vi "PI_GCS3_Configuration_Setup_Limits.vi"(0 "System no.":i32=1 min=1 step=1, 1 "Conn. Axes":string[](array[string]), 5 "error in":errorcluster) -> (14 "Positive Limit":dbl[](array[numeric]) format="%.6f", 16 "Negative Limit":dbl[](array[numeric]) format="%.6f", 19 "error out":errorcluster)   [LabVIEW 2026]
doc: "Gather positive and negative axes limits."
uses:
  SpecialCommand/ConfigurationMemoryType.ctl
panel:
  # "Gather positive and negative axes limits."
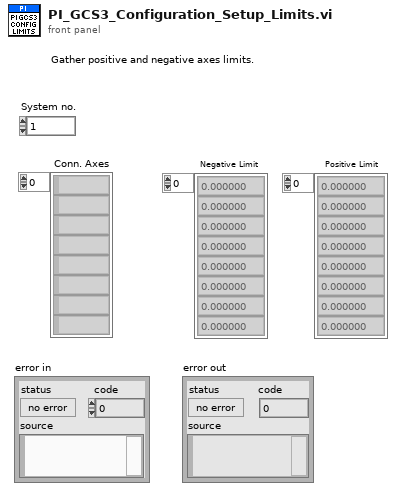
[diagram p1: front panel]
types:
  T1 = typedef "ConfigurationMemoryType.ctl" = enum16{"RAM", "TMP", "FLASH"}
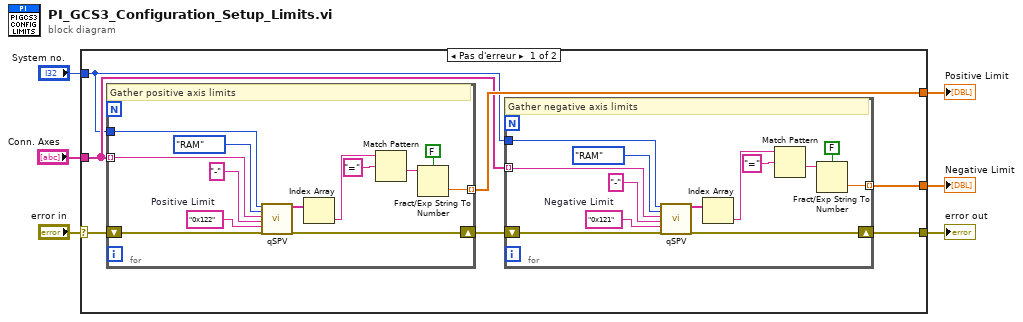
[diagram p0: block diagram]
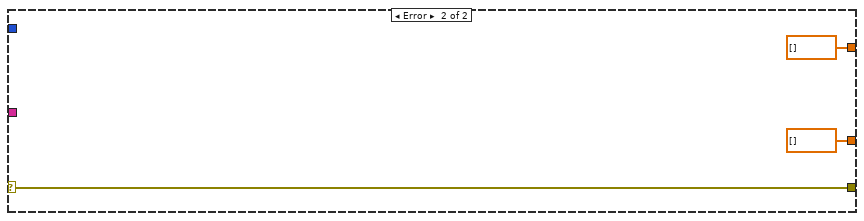
[diagram p2: hidden frame]
diagram:
  n1 = case shown="Pas d'erreur" "error in" {
    selector: "error in" -> [w13 w42]
    tunnel: [w8 w42] -> w5
    tunnel: "Conn. Axes" -> [w10 _]
    tunnel: "System no." -> [w9 _]
    tunnel: [w7 dbl[] [] ("Negative Limit")] -> w2
    tunnel: [w12 dbl[] [] ("Negative Limit")] -> w1
    frame No Error {
      n2 = for {
        shift-right: [w39] -> w11
        shift-left: w13 -> [w33]
        tunnel: w9 -> [w35]
        tunnel: w10 -> [w37] mode=indexing
        tunnel: [w32] -> w12 mode=indexing
        w38 = "0x122"  # Positive Limit
        # "Gather positive axis limits"
        n3 = call "qSPV.vi"("System no."=w35, "Target Memory Type"=ConfigurationMemoryType."RAM", "ContainerUnit"=w37, "FunctionUnit"="-", "ParameterID"=w38, "error in"=w33) -> ("Values"=w30:string[], "error out"=w39:errorcluster)  [unwired: 12 in]
        n4 = Index Array(array=w30) -> (element=w29:string)  [unwired: 1 in]
        n5 = Match Pattern(string=w29, regular expression="=") -> (after substring=w28:string)  [unwired: 1 in, 3 out]
        n6 = Fract/Exp String To Number(use system decimal point (T)=FALSE, string=w28) -> (number=w32:dbl)  [unwired: 2 in, 1 out]
      }
      n7 = for {
        shift-right: [w20] -> w8
        shift-left: w11 -> [w25]
        tunnel: w9 -> [w21]
        tunnel: w10 -> [w23] mode=indexing
        tunnel: [w19] -> w7 mode=indexing
        w26 = "0x121"  # Negative Limit
        # "Gather negative axis limits"
        n8 = call "qSPV.vi"("System no."=w21, "Target Memory Type"=ConfigurationMemoryType."RAM", "ContainerUnit"=w23, "FunctionUnit"="-", "ParameterID"=w26, "error in"=w25) -> ("Values"=w16:string[], "error out"=w20:errorcluster)  [unwired: 12 in]
        n9 = Index Array(array=w16) -> (element=w17:string)  [unwired: 1 in]
        n10 = Match Pattern(string=w17, regular expression="=") -> (after substring=w15:string)  [unwired: 1 in, 3 out]
        n11 = Fract/Exp String To Number(use system decimal point (T)=FALSE, string=w15) -> (number=w19:dbl)  [unwired: 2 in, 1 out]
      }
    }
    frame Error {
    }
  }
  "error out" <- w5
  "Negative Limit" <- w2
  "Positive Limit" <- w1
